vi "controlEotOutputDeactive.vi"(7 "Set":bool, 8 "error in":errorcluster, 9 "enable EOT in":bool=TRUE, 10 "axis in":u8, 11 "connection ID":refnum<k5>) -> (0 "error out":errorcluster, 1 "enable EOT out":bool=TRUE, 2 "axis out":u8, 3 "connection ID":refnum<k5>)   [LabVIEW 2016]
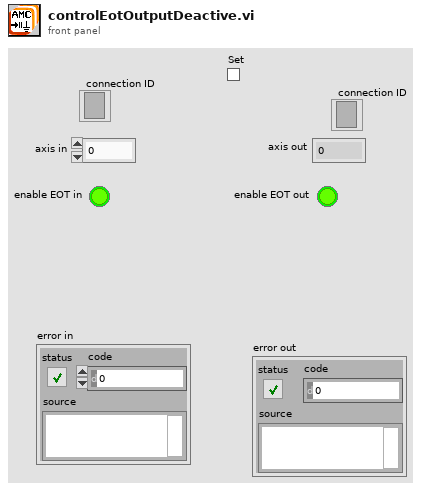
[diagram p1: front panel]
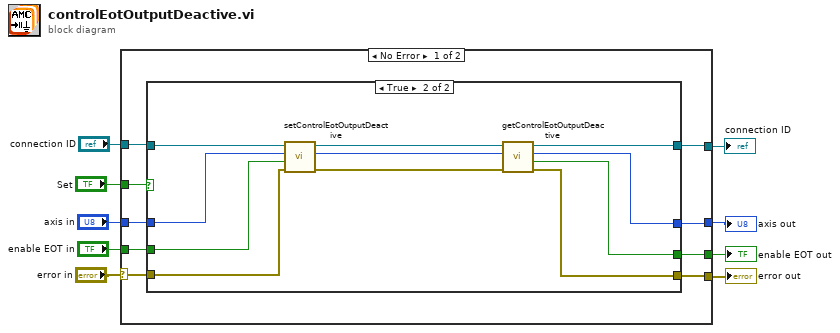
[diagram p0: block diagram]
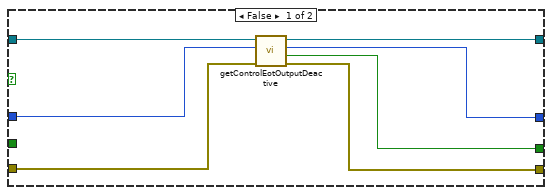
[diagram p2: hidden frame]
diagram:
  n1 = case shown="No Error" "error in" {
    selector: "error in" -> [w10 w40]
    tunnel: "axis in" -> [w16 w38]
    tunnel: [w11 w40] -> w8
    tunnel: [w13 w38] -> w7
    tunnel: "Set" -> [w17 _]
    tunnel: [w12 w39] -> w5
    tunnel: "enable EOT in" -> [w15 w39]
    tunnel: [w14 w37] -> w3
    tunnel: "connection ID" -> [w18 w37]
    frame No Error {
      n2 = case shown="True" w17 {
        tunnel: [w24 w28] -> w14
        tunnel: w18 -> [w25 w36]
        tunnel: w16 -> [w21 w35]
        tunnel: [w22 w27] -> w13
        tunnel: [w23 w26] -> w12
        tunnel: [w19 w31] -> w11
        tunnel: w15 -> [_ w33]
        tunnel: w10 -> [w20 w34]
        frame False {
          n3 = call "getControlEotOutputDeactive.vi"("error in"=w20, "axis"=w21, "connection ID"=w25) -> ("error out"=w19:errorcluster, "boolean"=w23:bool, "axis_out"=w22:i32, "connection ID"=w24:refnum<k5>)  [unwired: 5 in]
        }
        frame True {
          n4 = call "setControlEotOutputDeactive.vi"("error in"=w34, "enable"=w33, "axis"=w35, "connection ID"=w36) -> ("error out"=w32:errorcluster, "axis_out"=w29:i32, "connection ID"=w30:refnum<k5>)  [unwired: 5 in]
          n5 = call "getControlEotOutputDeactive.vi"("error in"=w32, "axis"=w29, "connection ID"=w30) -> ("error out"=w31:errorcluster, "boolean"=w26:bool, "axis_out"=w27:i32, "connection ID"=w28:refnum<k5>)  [unwired: 5 in]
        }
      }
    }
    frame Error {
    }
  }
  "error out" <- w8
  "axis out" <- w7
  "enable EOT out" <- w5
  "connection ID" <- w3
